vi "Log Fault.vi"(7 "max size (in bytes)":i64=50000, 8 "error in":errorcluster, 10 "Error String":string, 11 "Path In":path) -> (0 "error out":errorcluster)   [LabVIEW 2014]
doc: "This VI logs XML-RPC faults returned to the server to file"
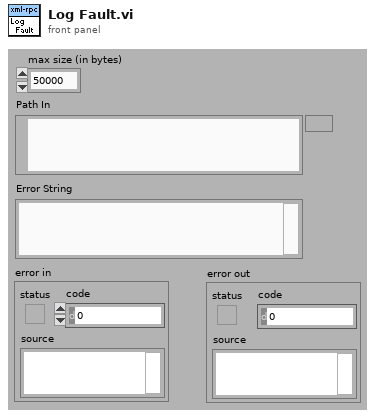
[diagram p1: front panel]
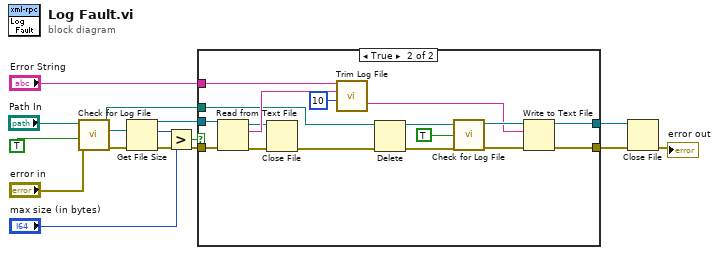
[diagram p0: block diagram]
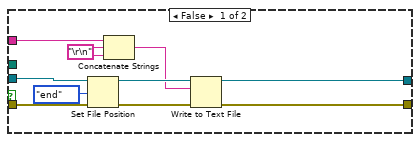
[diagram p2: hidden frame]
diagram:
  n1 = call "Check for Log File.vi"("error in"="error in", "Open File?"=TRUE, "Path In"="Path In") -> ("error out"=w7:errorcluster, "refnum out"=w8:refnum<file>, "Path Out"=w1:path)  [unwired: 6 in]
  n2 = Get File Size(file=w8, error in=w7) -> (refnum out=w3:refnum<file>, size (in bytes)=w5:i64, 0:w2:errorcluster)
  n3 = Greater?(x=w5, y="max size (in bytes)") -> (0:w6:bool)
  n4 = case shown="True" w6 {
    tunnel: [w25 w39] -> w12
    tunnel: [w24 w40] -> w11
    tunnel: "Error String" -> [w20 w38]
    tunnel: w3 -> [w17 w41]
    tunnel: w2 -> [w16 w42]
    tunnel: w1 -> [_ w31]
    frame False {
      w18 = "\r\n"
      n5 = Set File Position(refnum=w17, from (0:start)=enum16{"start", "end", "current"}."end", error in=w16) -> (refnum out=w22:refnum<file>, error out=w21:errorcluster)  [unwired: 1 in]
      n6 = Concatenate Strings(w20, w18, w18) -> (w19:string)
      n7 = Write to Text File(file (use dialog)=w22, text=w19, error in=w21) -> (refnum out=w24:refnum<file>, error out=w25:errorcluster)  [unwired: 1 in, 1 out]
    }
    frame True {
      n8 = Read from Text File(file (use dialog)=w41, error in=w42) -> (refnum out=w27:refnum<file>, text=w37:string, error out=w28:errorcluster)  [unwired: 2 in, 1 out]
      n9 = Close File(refnum=w27, error in=w28) -> (error out=w26:errorcluster)  [unwired: 1 out]
      n10 = call "Trim Log File.vi"("Trim n entries"=10, "Fault Log Contents"=w37, "Fault Message"=w38) -> ("Trimmed Fault Log"=w33:string)  [unwired: 8 in]
      n11 = Delete(path (use dialog)=w31, error in=w26) -> (deleted path=w30:path, error out=w32:errorcluster)  [unwired: 3 in, 1 out]
      n12 = call "Check for Log File.vi"("error in"=w32, "Open File?"=TRUE, "Path In"=w30) -> ("error out"=w34:errorcluster, "refnum out"=w35:refnum<file>)  [unwired: 6 in, 1 out]
      n13 = Write to Text File(file (use dialog)=w35, text=w33, error in=w34) -> (refnum out=w40:refnum<file>, error out=w39:errorcluster)  [unwired: 1 in, 1 out]
    }
  }
  n14 = Close File(refnum=w11, error in=w12) -> (error out=→"error out":errorcluster)  [unwired: 1 out]
